vi "Tenerowicz_Host_C.vi"() -> ()   [LabVIEW 2023]
panel:
  out "Waveform Graph":dbl[](graph)
  in  "SignalSend":bool
  in  "Stop":bool
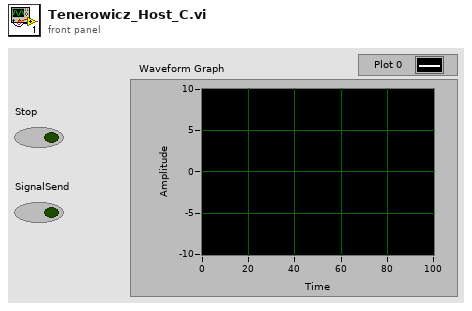
[diagram p1: front panel]
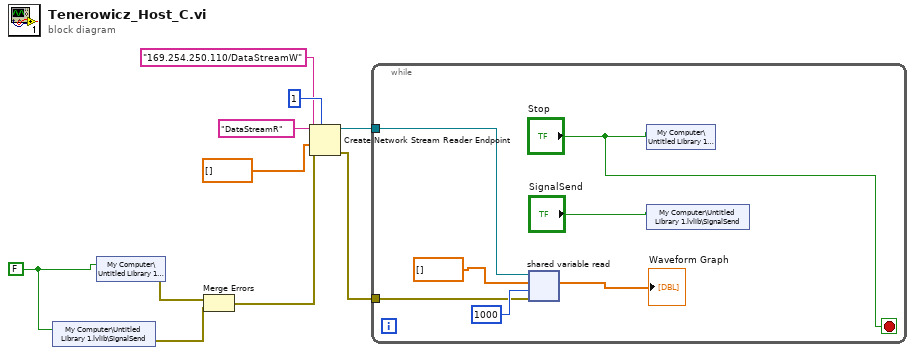
[diagram p0: block diagram]
diagram:
  w4 = FALSE ("Stop")
  n1 = shared-variable "My Computer\\Untitled Library 1.lvlib\\SignalSend"(w4) -> (error out=w6:errorcluster)  [unwired: 1 in]
  n2 = shared-variable "My Computer\\Untitled Library 1.lvlib\\Stop"(w4) -> (error out=w3:errorcluster)  [unwired: 1 in]
  n3 = Merge Errors(w3, w6) -> (w5:errorcluster)
  n4 = Create Network Stream Reader Endpoint(7:1 ("reader buffer size"), 8:w5, 9:dbl[] [] ("type"), 10:"169.254.250.110/DataStreamW" ("writer url"), 11:"DataStreamR" ("reader name")) -> (0:w1:errorcluster, 3:w2:refnum<k21>)  [unwired: 2 in]
  n5 = while {
    tunnel: w2 -> [w12]
    tunnel: w1 -> [w11]
    stop <- "Stop" stop-if-true
    n6 = shared-variable-read(w12, w11, dbl[] [], 1000 ("timeout ms (-1)")) -> (→"Waveform Graph":dbl[])  [unwired: 3 out]
    n7 = shared-variable "My Computer\\Untitled Library 1.lvlib\\Stop"("Stop") -> ()  [unwired: 1 in, 1 out]
    n8 = shared-variable "My Computer\\Untitled Library 1.lvlib\\SignalSend"("SignalSend") -> ()  [unwired: 1 in, 1 out]
  }
